vi "CRYDelete Command Idx.vi"(11 "Command Idx In":i32) -> ()   [LabVIEW 2013]
uses:
  CRYNew View Global.vi
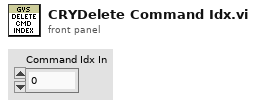
[diagram p1: front panel]
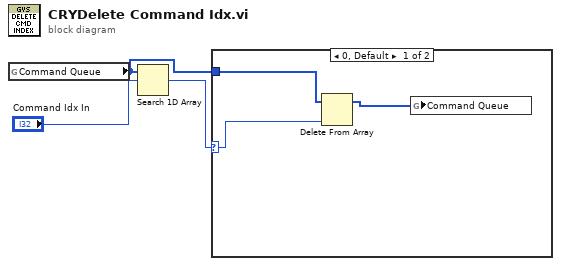
[diagram p0: block diagram]
diagram:
  n1 = global read "CRYNew View Global.vi" "Command Queue"() -> (w1:i32[])
  n2 = Search 1D Array(1D array=w1, element="Command Idx In") -> (index of element=w2:i32)  [unwired: 1 in]
  n3 = case shown="0, Default" w2 {
    selector: w2 -> [w5 _]
    tunnel: w1 -> [w6 _]
    frame 0, Default {
      n4 = Delete From Array(array=w6, index=w5) -> (array with subset deleted=w4:i32[])  [unwired: 1 in, 1 out]
      n5 = global write "CRYNew View Global.vi" "Command Queue"(w4) -> ()
    }
    frame -1 {
    }
  }
